vi "Get Measure And Log Message.vi"(11 "MyMessage":refnum<class "Channel Message.lvclass">) -> (1 "ackNeeded":bool, 2 "args":variant, 3 "command":string, 4 "id":u32)   [LabVIEW 2023, in "MeasureAndLogMessage.lvclass"]
uses:
  MeasureAndLogMessage.lvclass
  <vilib>/ChannelSupport/Channel Message/Channel Message.lvclass
  <vilib>/ChannelSupport/Channel Message/Channel Message.lvclass/Channel Message.ctl
  MeasureAndLogMessage.lvclass/MeasureAndLogMessage.ctl
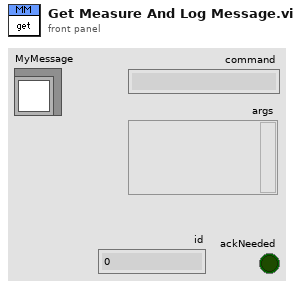
[diagram p1: front panel]
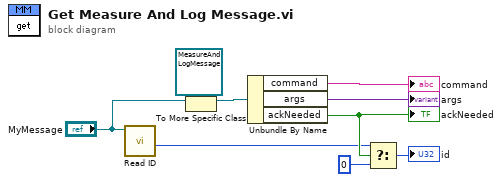
[diagram p0: block diagram]
diagram:
  n1 = call <vilib>:"Read ID.vi"("Channel Message in"="MyMessage") -> ("id"=w4:u32)  [unwired: 10 in]
  n2 = To More Specific Class(target class=refnum<class "MeasureAndLogMessage.lvclass"> refnum ("MyMessage.lvclass"), reference="MyMessage") -> (specific class reference=w7:refnum<class "MeasureAndLogMessage.lvclass">)  [unwired: 1 in, 1 out]
  n3 = Unbundle By Name(w7) -> ("command"=→"command":string, "args"=→"args":variant, "ackNeeded"=w5:bool)
  "ackNeeded" <- w5
  n4 = Select(t=w4, s=w5, f=u32 0) -> (s? t:f=→"id":u32)
